vi "Stream Split Character Match RegExp Std Out.vi"(8 "error in (no error)":errorcluster, 11 "Custom Regex in":refnum<class "Custom Regex.lvclass">) -> (0 "error out":errorcluster, 2 "Stream Split Character Match RegExp Std Out":string)   [LabVIEW 2024, in "serenial.io-ase.test.lvlib" / "Custom Regex.lvclass"]
uses:
  Custom Regex.lvclass
  Custom Regex.lvclass/Custom Regex.ctl
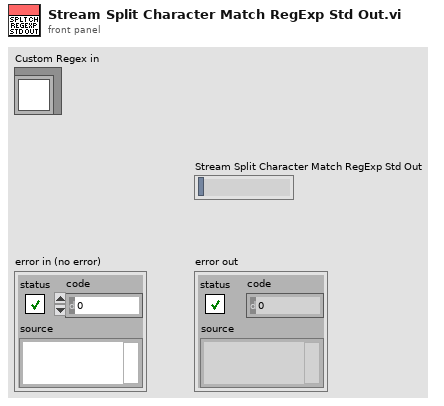
[diagram p1: front panel]
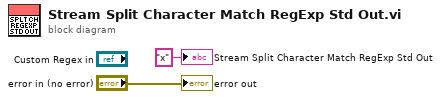
[diagram p0: block diagram]
diagram:
  "error out" <- "error in (no error)"
  "Stream Split Character Match RegExp Std Out" <- "x" ("Stream Split Character Match RegExp Std Out")
